vi "Generate Image.vi"() -> ()   [LabVIEW 2016, in "Map.lvclass"]
uses:
  Map.lvclass
  Grid/Grid.lvclass
panel:
  out "Value":picture
  out "Array":picture[][](array[picture])
  in  "Map.lvclass":refnum<class "Map.lvclass">
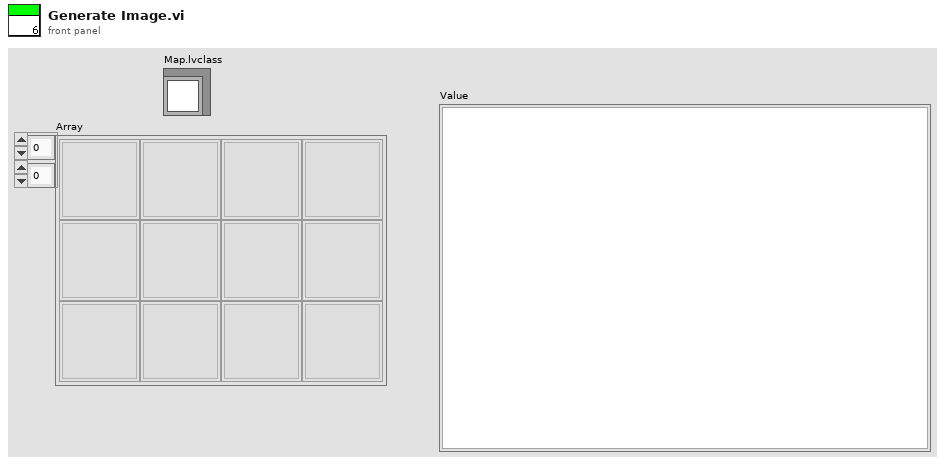
[diagram p1: front panel]
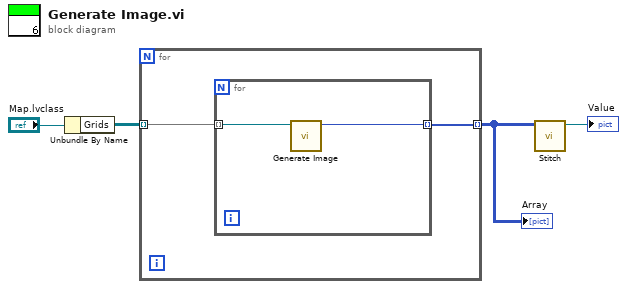
[diagram p0: block diagram]
diagram:
  n1 = Unbundle By Name("Map.lvclass") -> ("Grids"=w3:refnum<class "Grid.lvclass">[][])
  n2 = for {
    tunnel: w3 -> [w6] mode=indexing
    tunnel: [w5] -> w2 mode=indexing
    n3 = for {
      tunnel: w6 -> [w8] mode=indexing
      tunnel: [w7] -> w5 mode=indexing
      n4 = call "Generate Image.vi"("Grid.lvclass"=w8) -> ("new picture"=w7:picture)  [unwired: 10 in]
    }
  }
  "Array" <- w2
  n5 = call "Stitch.vi"("Map.lvclass"=w2) -> ("output cluster"=→"Value":refnum<class "Map.lvclass">)  [unwired: 9 in, 1 out]
